vi "obis set power.vi"(8 "error in":errorcluster, 10 "Power":dbl, 11 "Serial Port":refnum<visa-resource-name>) -> (0 "error out":errorcluster, 3 "Serial Port 2":refnum<visa-resource-name>)   [LabVIEW 2023, in "Coherent Laser.lvlib"]
uses:
  <vilib>/Utility/error.llb/Trim Whitespace One-Sided.vi
  Coherent Laser.lvlib
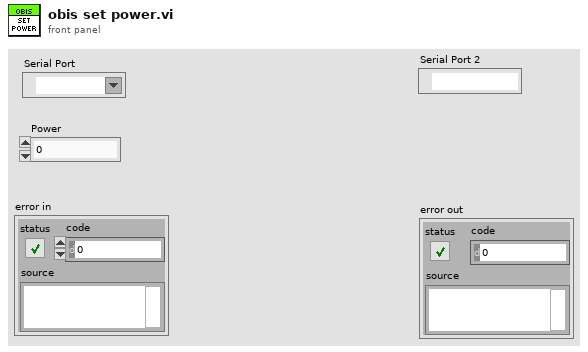
[diagram p1: front panel]
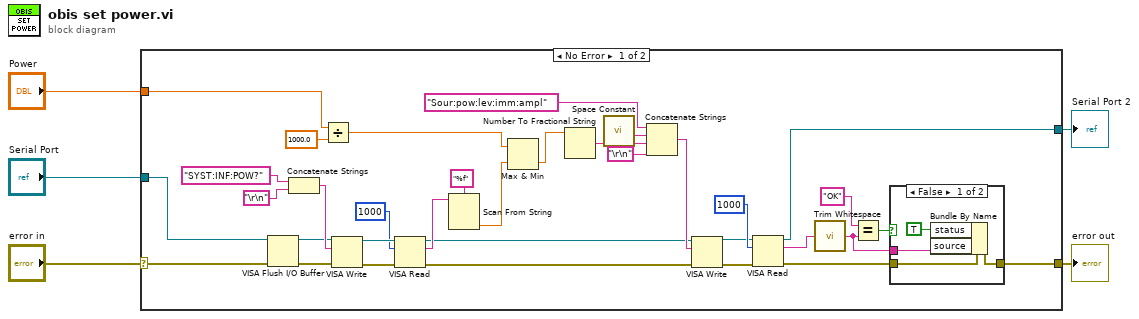
[diagram p0: block diagram]
diagram:
  n1 = case shown="No Error" "error in" {
    selector: "error in" -> [w14 w46]
    tunnel: [w19 w46] -> w4
    tunnel: "Serial Port" -> [w12 w45]
    tunnel: "Power" -> [w18 _]
    tunnel: [w17 w45] -> w1
    frame No Error {
      n2 = VISA Flush I/O Buffer(VISA resource name=w12, error in (no error)=w14) -> (VISA resource name out=w11:refnum<visa-resource-name>, error out=w13:errorcluster)  [unwired: 1 in]
      n3 = Concatenate Strings("SYST:INF:POW?" ("write buffer"), "\r\n") -> (w23:string)
      n4 = Divide(x=w18, y=1000.0) -> (x/y=w7:dbl)
      n5 = VISA Write(VISA resource name=w11, write buffer=w23, error in (no error)=w13) -> (VISA resource name out=w24:refnum<visa-resource-name>, error out=w25:errorcluster)  [unwired: 1 out]
      n6 = VISA Read(VISA resource name=w24, byte count=u32 1000, error in (no error)=w25) -> (VISA resource name out=w10:refnum<visa-resource-name>, read buffer=w16:string, error out=w9:errorcluster)  [unwired: 1 out]
      n7 = Scan From String(format string="%f", input string=w16) -> (output 1=w6:dbl)  [unwired: 3 in, 3 out]
      n8 = Max & Min(x=w7, y=w6) -> (min(x,y)=w8:dbl)  [unwired: 1 out]
      n9 = Number To Fractional String(number=w8) -> (F-format string=w39:string)  [unwired: 3 in]
      n10 = call <vilib>:"Space Constant.vi"() -> ("String"=w38:string)
      n11 = Concatenate Strings("Sour:pow:lev:imm:ampl" ("write buffer"), w38, w39, "\r\n") -> (w37:string)
      n12 = VISA Write(VISA resource name=w10, write buffer=w37, error in (no error)=w9) -> (VISA resource name out=w31:refnum<visa-resource-name>, error out=w32:errorcluster)  [unwired: 1 out]
      n13 = VISA Read(VISA resource name=w31, byte count=u32 1000, error in (no error)=w32) -> (VISA resource name out=w17:refnum<visa-resource-name>, read buffer=w30:string, error out=w28:errorcluster)  [unwired: 1 out]
      n14 = call <vilib>:"Trim Whitespace.vi"("string"=w30) -> ("trimmed string"=w26:string)  [unwired: 1 in]
      n15 = Equal?(x="OK", y=w26) -> (x = y?=w27:bool)
      n16 = case shown="False" w27 {
        tunnel: w28 -> [w42 w44]
        tunnel: [w43 w44] -> w19
        tunnel: w26 -> [w41 _]
        frame False {
          n17 = Bundle By Name(cluster=w42, "status"=TRUE, "source"=w41) -> (w43:errorcluster)
        }
        frame True {
        }
      }
    }
    frame Error {
    }
  }
  "error out" <- w4
  "Serial Port 2" <- w1
